vi "Sim_Yoke_Shin_TP059851_SPCC_Assignment.vi"() -> ()   [LabVIEW 2020]
uses:
  EnumControl.ctl
panel:
  in  "Enter":bool
  in  "User Input":string
  in  "Card Simulator":bool
  in  "Right Buttons":T1
  out "Right Menu":T2
  in  "Left Buttons":T3
  out "Left Menu":T4
  out "ATM Messages":string
  out "User ID":string
  out "Main Menu message":string
  out "Login":errorcluster
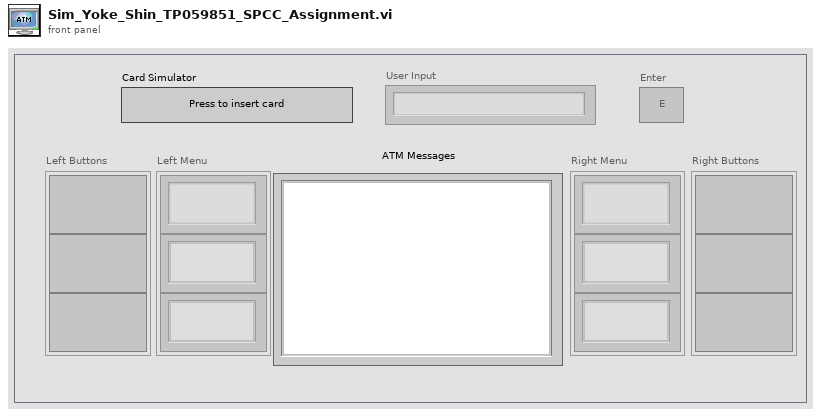
[diagram p1: front panel]
types:
  T1 = cluster{"Right 1 btn":bool, "Right 2 btn":bool, "Right 3 btn":bool}
  T2 = cluster{"Right 1 lbl":string, "Right 2 lbl":string, "Right 3 lbl":string}
  T3 = cluster{"Left 1 btn":bool, "Left 2 btn":bool, "Left 3 btn":bool}
  T4 = cluster{"Left 1 lbl":string, "Left 2 lbl":string, "Left 3 lbl":string}
  T5 = typedef "EnumControl.ctl" = enum16{"Idle", "Insert card", "Login click", "Validate Account", "Active Main Page", "Menu btn event", "Balance", "Deposit", "Withdraw", "Fast Cash", "Terminate"}
  T6 = enum8{"Enabled", "Disabled", "Disabled and Grayed Out"}
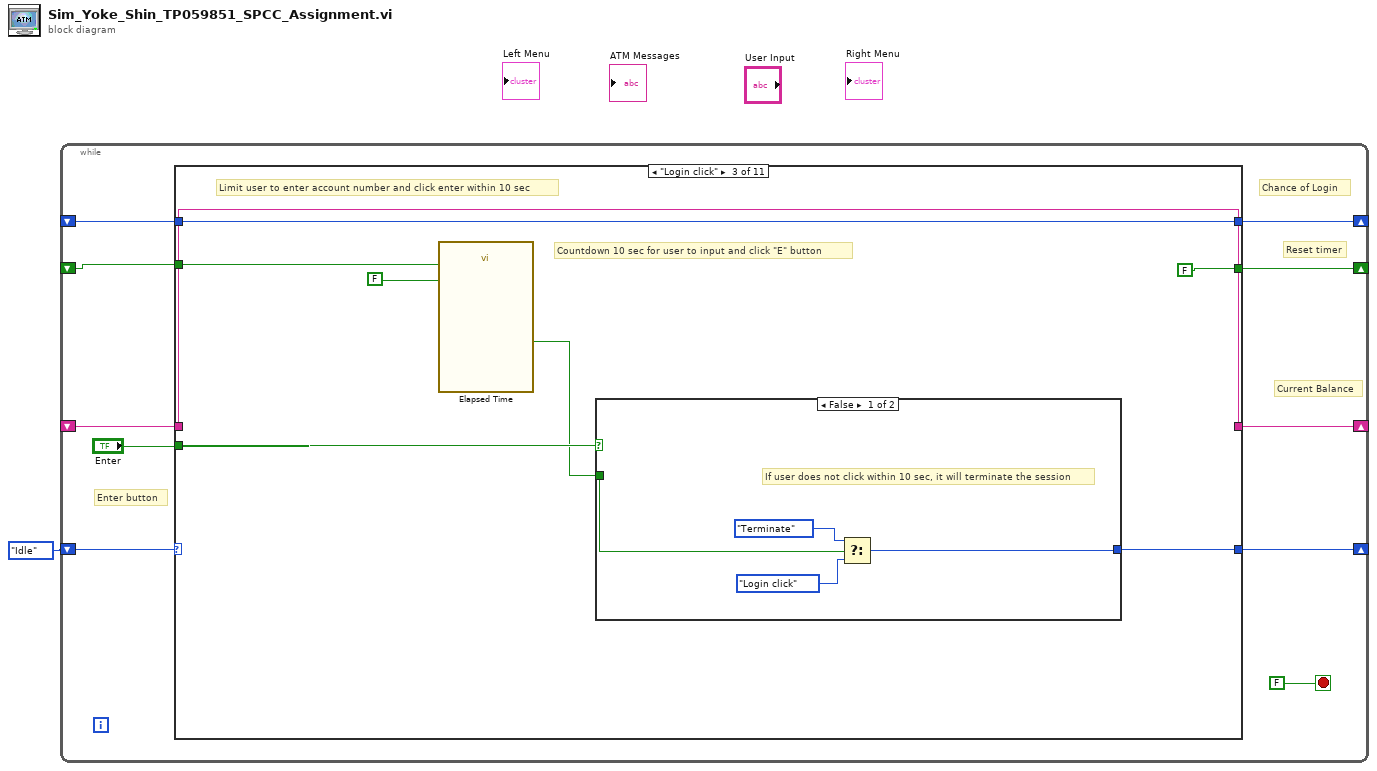
[diagram p0: block diagram]
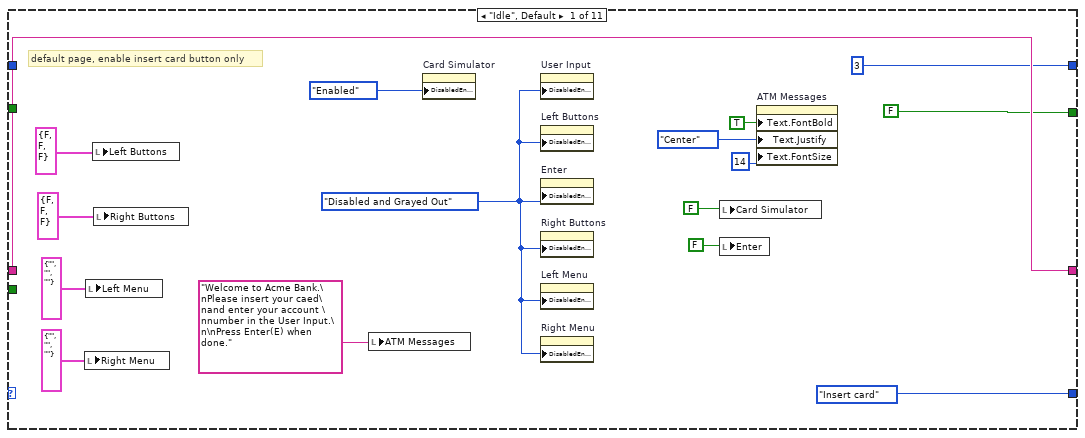
[diagram p2: hidden frame]
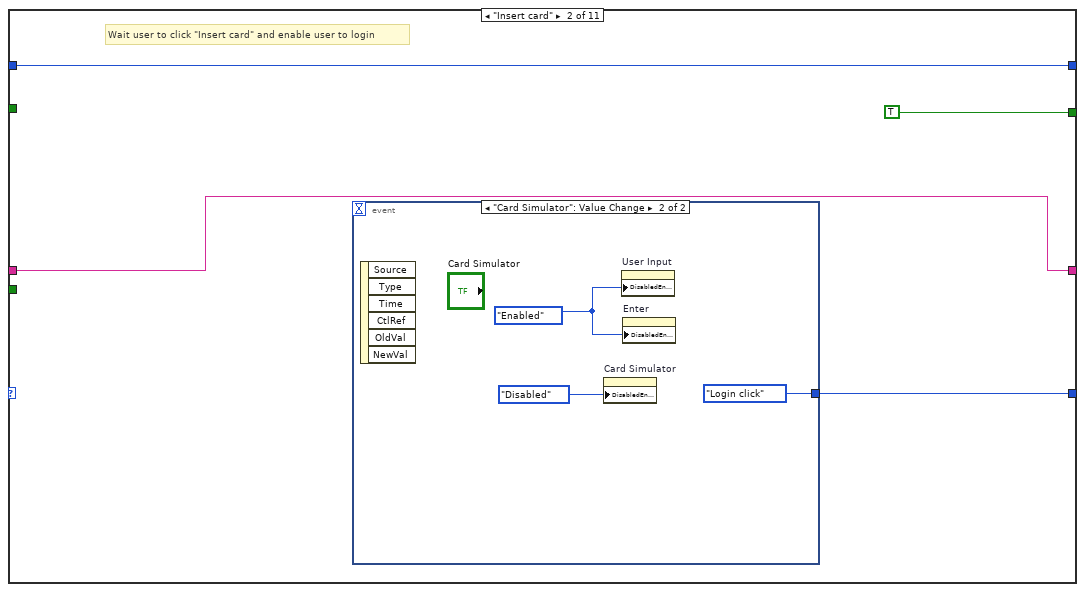
[diagram p3: hidden frame]
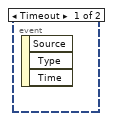
[diagram p4: hidden frame]
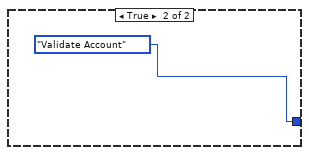
[diagram p5: hidden frame]
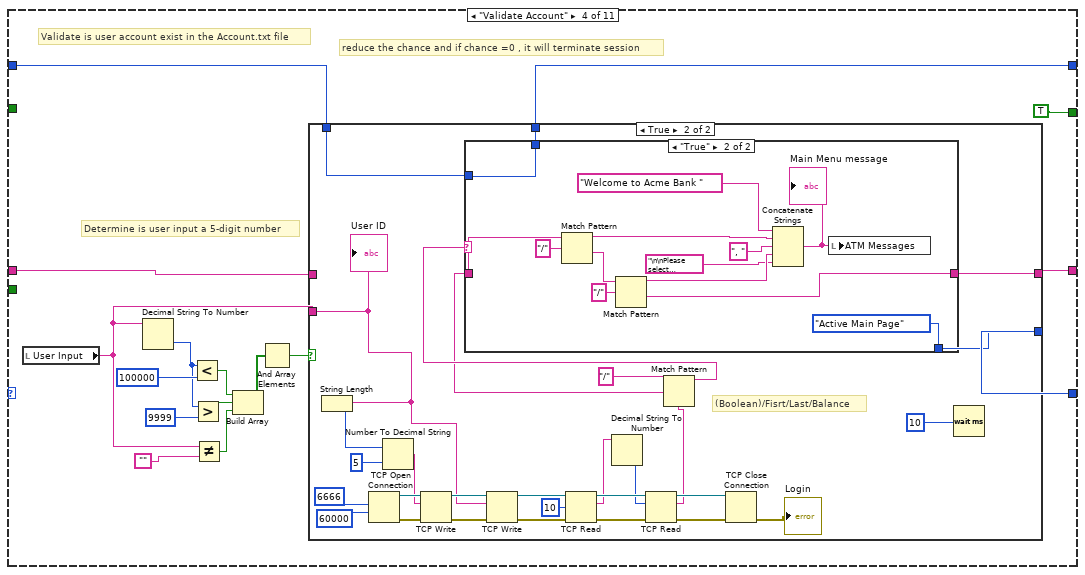
[diagram p6: hidden frame]
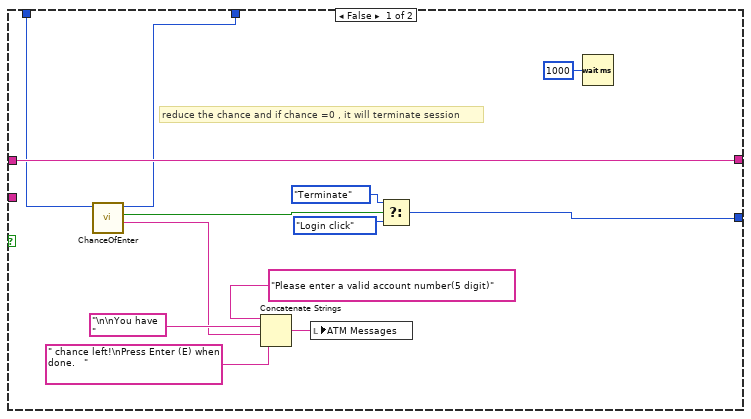
[diagram p7: hidden frame]
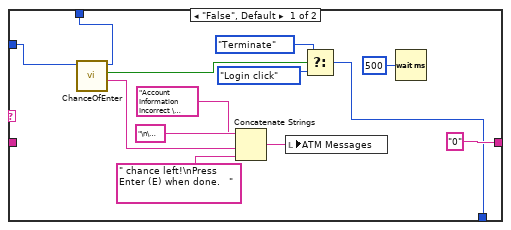
[diagram p8: hidden frame]
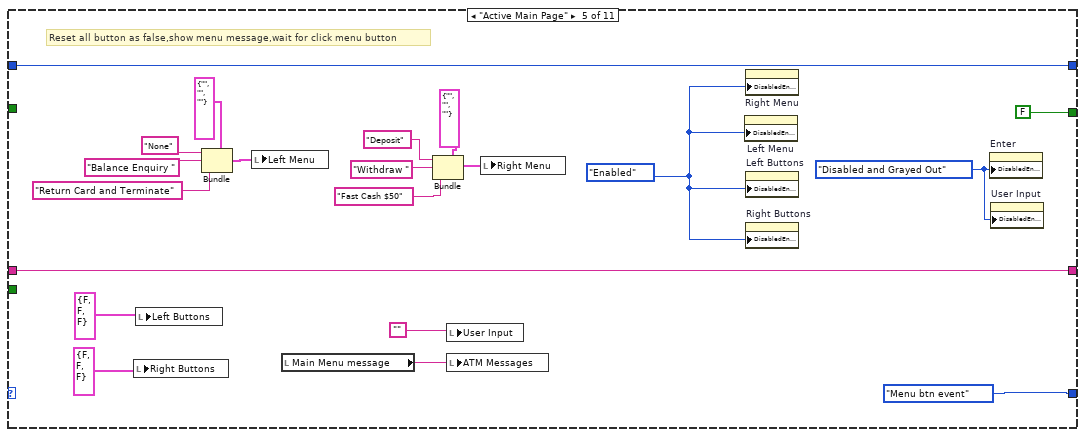
[diagram p9: hidden frame]
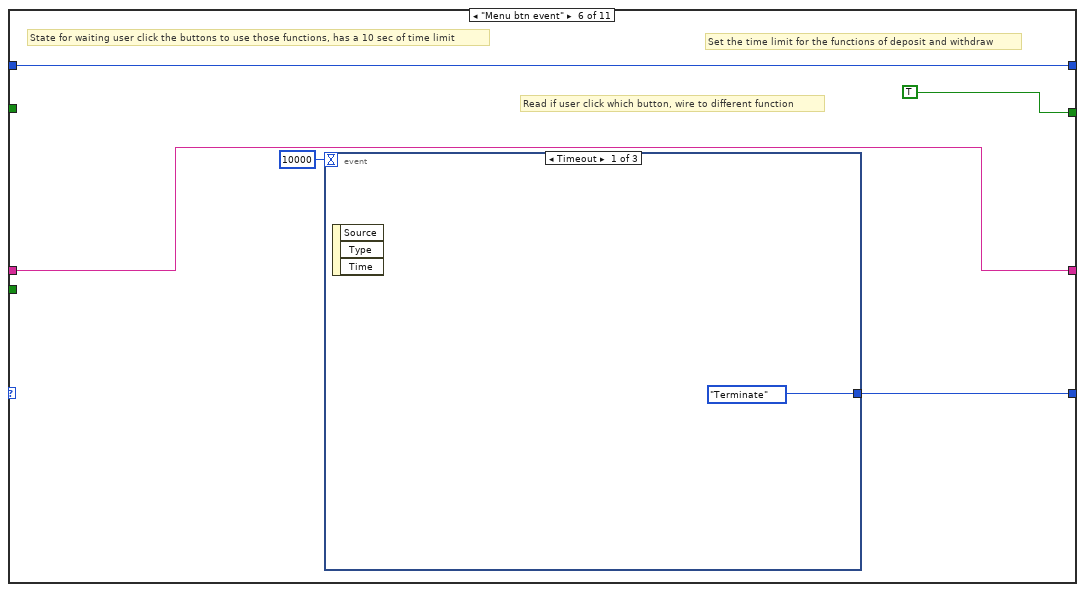
[diagram p10: hidden frame]
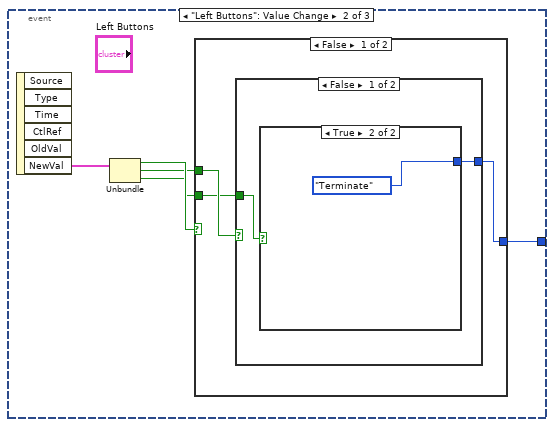
[diagram p11: hidden frame]
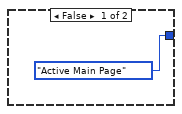
[diagram p12: hidden frame]
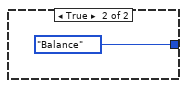
[diagram p13: hidden frame]
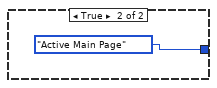
[diagram p14: hidden frame]
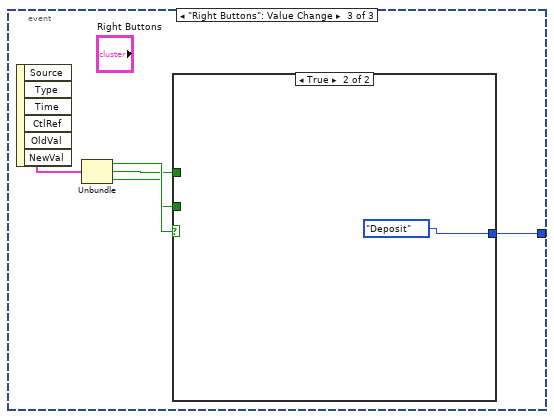
[diagram p15: hidden frame]
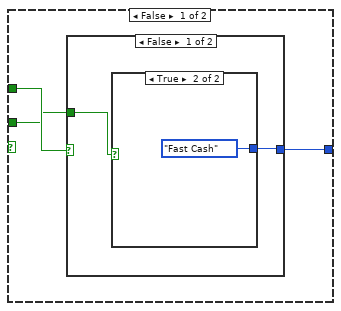
[diagram p16: hidden frame]
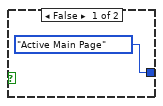
[diagram p17: hidden frame]
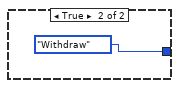
[diagram p18: hidden frame]
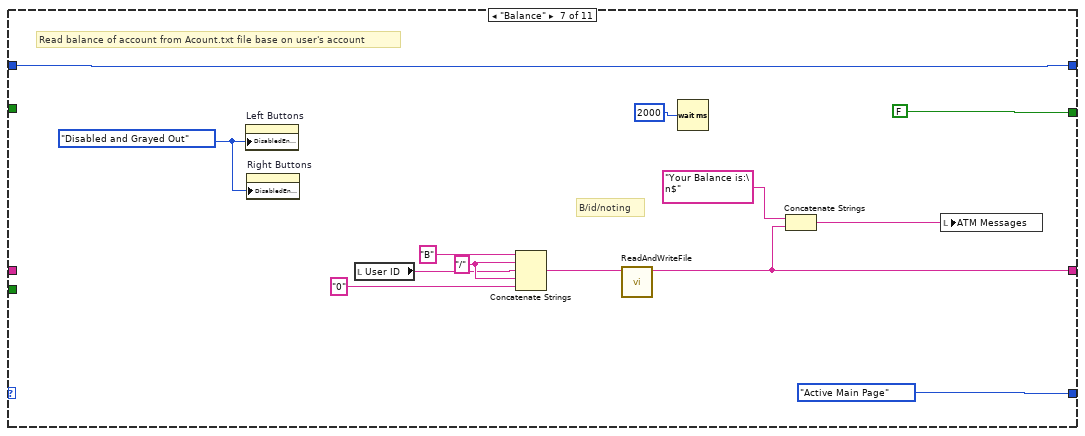
[diagram p19: hidden frame]
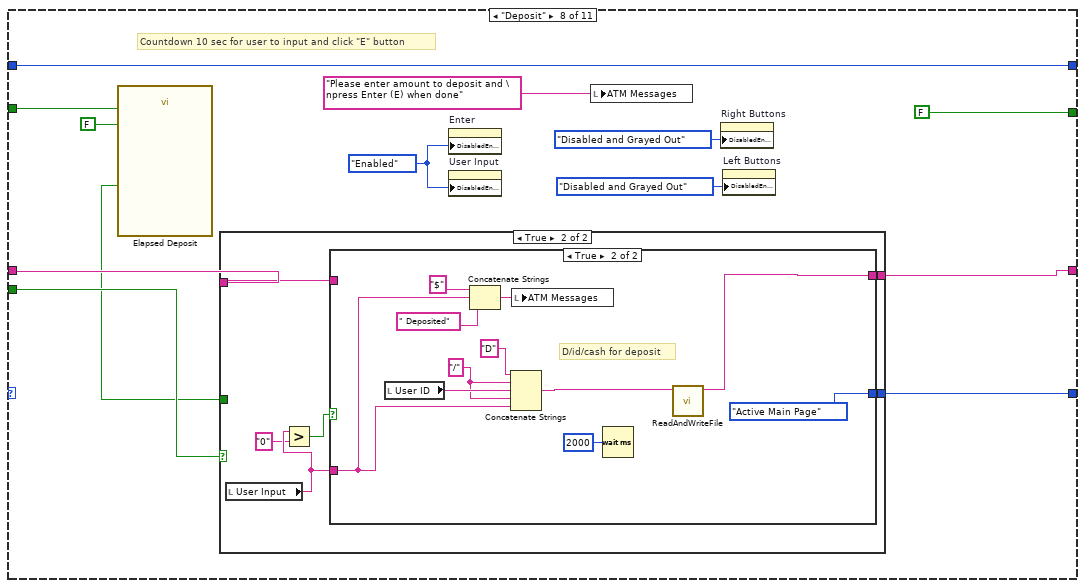
[diagram p20: hidden frame]
diagram:
  n1 = while {
    shift-right: [w9] -> _
    shift-left: EnumControl."Idle" ("Enum") -> [w11]
    shift-right: [w7] -> _
    shift-left: _ -> [w8]
    shift-right: [w4] -> _
    shift-left: _ -> [w5]
    shift-right: [w3] -> _
    shift-left: _ -> [w2]
    stop <- FALSE stop-if-true
    # "Enter button"
    # "Reset timer"
    # "Chance of Login"
    # "Current Balance"
    n2 = case shown="\"Login click\"" w11 {
      tunnel: [EnumControl."Insert card" ("Enum") w31 w41 w63 EnumControl."Menu btn event" ("Enum") w156 EnumControl."Active Main Page" ("Enum") w211 w250 w299 EnumControl."Idle" ("Enum")] -> w9
      tunnel: "Enter" -> [_ _ w42 _ _ _ _ w209 w248 _ _]
      tunnel: [w15 w30 w40 w62 w135 w155 w186 w206 w245 w297 w328] -> w7
      tunnel: w8 -> [w15 w30 w40 w55 w135 w155 _ w207 w246 w294 w328]
      tunnel: w5 -> [_ _ w37 _ _ _ _ w201 w240 _ _]
      tunnel: [FALSE TRUE FALSE TRUE FALSE TRUE FALSE FALSE FALSE FALSE FALSE] -> w4
      tunnel: [3 w28 w35 w60 w133 w152 w189 w199 w238 w295 3] -> w3
      tunnel: w2 -> [_ w28 w35 w61 w133 w152 w189 w199 w238 w295 _]
      frame "Idle", Default {
        w18 = T6."Disabled and Grayed Out" ("Disabled")
        # "default page, enable insert card button only"
        n3 = local write "Right Menu"(T2 {"Right 1 lbl"="", "Right 2 lbl"="", "Right 3 lbl"=""} ("right lbl")) -> ()
        n4 = local write "Left Menu"(T4 {"Left 1 lbl"="", "Left 2 lbl"="", "Left 3 lbl"=""} ("left lbl")) -> ()
        n5 = local write "Left Buttons"(T3 {"Left 1 btn"=FALSE, "Left 2 btn"=FALSE, "Left 3 btn"=FALSE} ("Left btn")) -> ()
        n6 = local write "Right Buttons"(T1 {"Right 1 btn"=FALSE, "Right 2 btn"=FALSE, "Right 3 btn"=FALSE} ("right btn")) -> ()
        n7 = local write "ATM Messages"("Welcome to Acme Bank.\nPlease insert your caed\nand enter your account \nnumber in the User Input.\n\nPress Enter(E) when done." ("ATM Messages")) -> ()
        n8 = property on="Card Simulator" class="Bool (strict)"("DisabledEnum"=T6."Enabled" ("Disabled")) -> ()  [unwired: 2 in, 2 out]
        n9 = property on="User Input" class="Str"("DisabledEnum"=w18) -> ()  [unwired: 2 in, 2 out]
        n10 = property on="Left Buttons" class="Clust (strict)"("DisabledEnum"=w18) -> ()  [unwired: 2 in, 2 out]
        n11 = property on="Enter" class="Bool (strict)"("DisabledEnum"=w18) -> ()  [unwired: 2 in, 2 out]
        n12 = property on="Right Buttons" class="Clust (strict)"("DisabledEnum"=w18) -> ()  [unwired: 2 in, 2 out]
        n13 = property on="Left Menu" class="Clust (strict)"("DisabledEnum"=w18) -> ()  [unwired: 2 in, 2 out]
        n14 = property on="Right Menu" class="Clust (strict)"("DisabledEnum"=w18) -> ()  [unwired: 2 in, 2 out]
        n15 = local write "Card Simulator"(FALSE ("Card Simulator")) -> ()
        n16 = local write "Enter"(FALSE ("Enter")) -> ()
        n17 = property on="ATM Messages" class="Str"("Text.FontBold"=TRUE ("Text.Font:Bold"), "Text.Justify"=enum16{"Left", "Center", "Right"}."Center" ("Text.Justification"), "Text.FontSize"=u32 14 ("Text.Font:Size")) -> ()  [unwired: 2 in, 2 out]
      }
      frame "Insert card" {
        # "Wait user to click \"Insert card\" and enable user to login"
        n18 = event shown="[1] \"Card Simulator\": Value Change" {
          selector: _ -> [_ _]
          dyn-events: _ -> [_ _]
          timeout: _ -> [_ _]
          tunnel: [_ EnumControl."Login click" ("Enum")] -> w31
          event Timeout {
            n19 = event-data() -> ()  [unwired: 1 in, 3 out]
          }
          event "Card Simulator": Value Change {
            w34 = T6."Enabled" ("Disabled")
            n20 = event-data() -> ()  [unwired: 1 in, 6 out]
            n21 = property on="Card Simulator" class="Bool (strict)"("DisabledEnum"=T6."Disabled" ("Disabled")) -> ()  [unwired: 2 in, 2 out]
            n22 = property on="User Input" class="Str"("DisabledEnum"=w34) -> ()  [unwired: 2 in, 2 out]
            n23 = property on="Enter" class="Bool (strict)"("DisabledEnum"=w34) -> ()  [unwired: 2 in, 2 out]
          }
        }
      }
      frame "Login click" {
        # "Limit user to enter account number and click enter within 10 sec"
        # "Countdown 10 sec for user to input and click \"E\" button"
        n24 = call "Elapsed Time"("Reset"=w37, "Auto Reset"=FALSE) -> ("Time has Elapsed"=w39:bool)  [unwired: 10 in, 7 out]
        n25 = case shown="False" w42 {
          tunnel: [w44 EnumControl."Validate Account" ("Enum")] -> w41
          tunnel: w39 -> [w43 _]
          frame False {
            # "If user does not click within 10 sec, it will terminate the session"
            n26 = Select(t=EnumControl."Terminate" ("Enum"), s=w43, f=EnumControl."Login click" ("Enum")) -> (s? t:f=w44:T5)
          }
          frame True {
          }
        }
      }
      frame "Validate Account" {
        # "Validate is user account exist in the Account.txt file"
        # "Determine is user input a 5-digit number"
        # "reduce the chance and if chance =0 , it will terminate session"
        n27 = local read "User Input"() -> (w57:string)
        n28 = Decimal String To Number(string=w57) -> (number=w53:i32)  [unwired: 2 in, 1 out]
        n29 = Less?(x=w53, y=100000) -> (x < y?=w50:bool)
        n30 = Greater?(x=w53, y=9999) -> (0:w51:bool)
        n31 = Not Equal?(x=w57, y="") -> (x != y?=w52:bool)
        n32 = Build Array "Build Array"(w50, w51, w52) -> (w49:bool[])
        n33 = And Array Elements(Boolean array=w49) -> (logical AND=w48:bool)
        n34 = case shown="True" w48 {
          tunnel: w57 -> [_ w90]
          tunnel: [w70 w82] -> w63
          tunnel: [w69 w79] -> w62
          tunnel: w61 -> [w67 w78]
          tunnel: [w66 w77] -> w60
          tunnel: w55 -> [w69 _]
          frame False {
            # "reduce the chance and if chance =0 , it will terminate session"
            n35 = call "ChanceOfEnter.vi"("Numeric in"=w67) -> ("String"=w64:string, "Boolean"=w65:bool, "Numeric out"=w66:i32)  [unwired: 8 in]
            n36 = Concatenate Strings("Please enter a valid account number(5 digit)" ("ATM Messages"), "\n\nYou have " ("string"), w64, " chance left!\nPress Enter (E) when done.   " ("string")) -> (w76:string)
            n37 = local write "ATM Messages"(w76) -> ()
            n38 = Select(t=EnumControl."Terminate" ("Enum"), s=w65, f=EnumControl."Login click" ("Enum")) -> (s? t:f=w70:T5)
            n39 = Wait (ms)(milliseconds to wait=u32 1000) -> ()  [unwired: 1 out]
          }
          frame True {
            # "(Boolean)/Fisrt/Last/Balance"
            n40 = String Length(string=w90) -> (length=w92:i32)
            n41 = TCP Open Connection(remote port or service name=u16 6666, timeout ms (60000)=60000) -> (connection ID=w97:refnum<k5>, error out=w105:errorcluster)  [unwired: 3 in]
            n42 = Number To Decimal String(number=w92, width (-)=i16 5) -> (decimal integer string=w91:string)
            n43 = TCP Write(connection ID=w97, data in=w91, error in (no error)=w105) -> (connection ID out=w96:refnum<k5>, error out=w104:errorcluster)  [unwired: 1 in, 1 out]
            n44 = TCP Write(connection ID=w96, data in=w90, error in (no error)=w104) -> (connection ID out=w95:refnum<k5>, error out=w103:errorcluster)  [unwired: 1 in, 1 out]
            n45 = TCP Read(connection ID=w95, bytes to read=10, error in (no error)=w103) -> (connection ID out=w94:refnum<k5>, data out=w88:string, error out=w102:errorcluster)  [unwired: 2 in]
            n46 = Decimal String To Number(string=w88) -> (number=w87:i32)  [unwired: 2 in, 1 out]
            n47 = TCP Read(connection ID=w94, bytes to read=w87, error in (no error)=w102) -> (connection ID out=w93:refnum<k5>, data out=w86:string, error out=w101:errorcluster)  [unwired: 2 in]
            n48 = Match Pattern(string=w86, regular expression="/") -> (before substring=w84:string, after substring=w83:string)  [unwired: 1 in, 2 out]
            n49 = case shown="\"True\"" w84 {
              tunnel: w83 -> [_ w131]
              tunnel: [w106 EnumControl."Active Main Page" ("Enum")] -> w82
              tunnel: ["0" ("data out") w120] -> w79
              tunnel: w78 -> [w113 w119]
              tunnel: [w110 w119] -> w77
              frame "False", Default {
                n50 = call "ChanceOfEnter.vi"("Numeric in"=w113) -> ("String"=w112:string, "Boolean"=w109:bool, "Numeric out"=w110:i32)  [unwired: 8 in]
                n51 = Concatenate Strings("Account Information Incorrect \nPlease Re-Enter Account Number. " ("ATM Messages"), "\n\nYou have " ("string"), w112, " chance left!\nPress Enter (E) when done.   " ("string")) -> (w116:string)
                n52 = local write "ATM Messages"(w116) -> ()
                n53 = Select(t=EnumControl."Terminate" ("Enum"), s=w109, f=EnumControl."Login click" ("Enum")) -> (s? t:f=w106:T5)
                n54 = Wait (ms)(milliseconds to wait=u32 500) -> ()  [unwired: 1 out]
              }
              frame "True" {
                n55 = Match Pattern(string=w131, regular expression="/") -> (before substring=w123:string, after substring=w125:string)  [unwired: 1 in, 2 out]
                n56 = Match Pattern(string=w125, regular expression="/") -> (before substring=w122:string, after substring=w120:string)  [unwired: 1 in, 2 out]
                n57 = Concatenate Strings("Welcome to Acme Bank " ("string"), w123, ", " ("string"), w122, "\n\nPlease select transaction by using the buttons. " ("string")) -> (w127:string)
                "Main Menu message" <- w127
                n58 = local write "ATM Messages"(w127) -> ()
              }
            }
            n59 = TCP Close Connection(connection ID=w93, error in (no error)=w101) -> (error out=→"Login":errorcluster)  [unwired: 1 in, 1 out]
            n60 = Wait (ms)(milliseconds to wait=u32 10) -> ()  [unwired: 1 out]
            "User ID" <- w90
          }
        }
      }
      frame "Active Main Page" {
        w141 = T6."Disabled and Grayed Out" ("Disabled")
        w138 = T6."Enabled" ("Disabled")
        # "Reset all button as false,show menu message,wait for click menu button"
        n61 = local write "Right Buttons"(T1 {"Right 1 btn"=FALSE, "Right 2 btn"=FALSE, "Right 3 btn"=FALSE} ("right btn")) -> ()
        n62 = local write "Left Buttons"(T3 {"Left 1 btn"=FALSE, "Left 2 btn"=FALSE, "Left 3 btn"=FALSE} ("Left btn")) -> ()
        n63 = Bundle(cluster=T2 {"Right 1 lbl"="", "Right 2 lbl"="", "Right 3 lbl"=""}, "Right 1 lbl"="None", "Right 2 lbl"="Balance Enquiry ", "Right 3 lbl"="Return Card and Terminate") -> (w147:T2)
        n64 = local write "Left Menu"(w147) -> ()
        n65 = local read "Main Menu message"() -> (w151:string)
        n66 = Bundle(cluster=T2 {"Right 1 lbl"="", "Right 2 lbl"="", "Right 3 lbl"=""}, "Right 1 lbl"="Deposit", "Right 2 lbl"="Withdraw ", "Right 3 lbl"="Fast Cash $50") -> (w142:T2)
        n67 = local write "User Input"("") -> ()
        n68 = local write "ATM Messages"(w151) -> ()
        n69 = local write "Right Menu"(w142) -> ()
        n70 = property on="Left Menu" class="Clust (strict)"("DisabledEnum"=w138) -> ()  [unwired: 2 in, 2 out]
        n71 = property on="Right Menu" class="Clust (strict)"("DisabledEnum"=w138) -> ()  [unwired: 2 in, 2 out]
        n72 = property on="Left Buttons" class="Clust (strict)"("DisabledEnum"=w138) -> ()  [unwired: 2 in, 2 out]
        n73 = property on="Right Buttons" class="Clust (strict)"("DisabledEnum"=w138) -> ()  [unwired: 2 in, 2 out]
        n74 = property on="Enter" class="Bool (strict)"("DisabledEnum"=w141) -> ()  [unwired: 2 in, 2 out]
        n75 = property on="User Input" class="Str"("DisabledEnum"=w141) -> ()  [unwired: 2 in, 2 out]
      }
      frame "Menu btn event" {
        # "State for waiting user click the buttons to use those functions, has a 10 sec of time limit"
        # "Set the time limit for the functions of deposit and withdraw"
        # "Read if user click which button, wire to different function"
        n76 = event shown="[0] Timeout" {
          selector: _ -> [_ _ _]
          dyn-events: _ -> [_ _ _]
          timeout: 10000 -> [_ _ _]
          tunnel: [EnumControl."Terminate" ("Enum") w160 w174] -> w156
          event Timeout {
            n77 = event-data() -> ()  [unwired: 1 in, 3 out]
          }
          event "Left Buttons": Value Change {
            n78 = event-data() -> ("NewVal"=w162:T3)  [unwired: 1 in, 5 out]
            n79 = Unbundle "Unbundle"(w162) -> ("Left 1 btn"=w161:bool, "Left 2 btn"=w159:bool, "Left 3 btn"=w158:bool)
            n80 = case shown="False" w161 {
              tunnel: [w164 EnumControl."Active Main Page" ("Enum")] -> w160
              tunnel: w159 -> [w165 _]
              tunnel: w158 -> [w163 _]
              frame False {
                n81 = case shown="False" w165 {
                  tunnel: [w166 EnumControl."Balance" ("Enum")] -> w164
                  tunnel: w163 -> [w167 _]
                  frame False {
                    n82 = case shown="True" w167 {
                      tunnel: [EnumControl."Active Main Page" ("Enum") EnumControl."Terminate" ("Enum")] -> w166
                      frame False {
                      }
                      frame True {
                      }
                    }
                  }
                  frame True {
                  }
                }
              }
              frame True {
              }
            }
          }
          event "Right Buttons": Value Change {
            n83 = event-data() -> ("NewVal"=w176:T1)  [unwired: 1 in, 5 out]
            n84 = Unbundle "Unbundle"(w176) -> ("Right 1 btn"=w175:bool, "Right 2 btn"=w173:bool, "Right 3 btn"=w172:bool)
            n85 = case shown="True" w175 {
              tunnel: [w178 EnumControl."Deposit" ("Enum")] -> w174
              tunnel: w173 -> [w179 _]
              tunnel: w172 -> [w177 _]
              frame False {
                n86 = case shown="False" w179 {
                  tunnel: [w180 EnumControl."Withdraw" ("Enum")] -> w178
                  tunnel: w177 -> [w181 _]
                  frame False {
                    n87 = case shown="True" w181 {
                      tunnel: [EnumControl."Active Main Page" ("Enum") EnumControl."Fast Cash" ("Enum")] -> w180
                      frame False {
                      }
                      frame True {
                      }
                    }
                  }
                  frame True {
                  }
                }
              }
              frame True {
              }
            }
          }
        }
      }
      frame "Balance" {
        w188 = T6."Disabled and Grayed Out" ("Disabled")
        w193 = "/" ("string")
        # "Read balance of account from Acount.txt file base on user's account"
        # "B/id/noting"
        n88 = property on="Left Buttons" class="Clust (strict)"("DisabledEnum"=w188) -> ()  [unwired: 2 in, 2 out]
        n89 = property on="Right Buttons" class="Clust (strict)"("DisabledEnum"=w188) -> ()  [unwired: 2 in, 2 out]
        n90 = local read "User ID"() -> (w192:string)
        n91 = Concatenate Strings("B" ("string"), w193, w192, w193, "0" ("string")) -> (w187:string)
        n92 = call "ReadAndWriteFile.vi"("String"=w187) -> ("data out"=w186:string)  [unwired: 10 in]
        n93 = Wait (ms)(milliseconds to wait=u32 2000) -> ()  [unwired: 1 out]
        n94 = Concatenate Strings("Your Balance is:\n$" ("ATM Messages"), w186) -> (w195:string)
        n95 = local write "ATM Messages"(w195) -> ()
      }
      frame "Deposit" {
        w210 = T6."Enabled" ("Disabled")
        # "Countdown 10 sec for user to input and click \"E\" button"
        n96 = call "Elapsed Deposit"("Reset"=w201, "Auto Reset"=FALSE) -> ("Time has Elapsed"=w200:bool)  [unwired: 10 in, 7 out]
        n97 = case shown="True" w209 {
          tunnel: [w212 w222] -> w211
          tunnel: w207 -> [w216 w221]
          tunnel: [w216 w220] -> w206
          tunnel: w200 -> [w215 _]
          frame False {
            n98 = Select(t=EnumControl."Terminate" ("Enum"), s=w215, f=EnumControl."Deposit" ("Enum")) -> (s? t:f=w212:T5)
          }
          frame True {
            n99 = local read "User Input"() -> (w219:string)
            n100 = Greater?(x=w219, y="0") -> (0:w217:bool)
            n101 = case shown="True" w217 {
              tunnel: [EnumControl."Active Main Page" ("Enum") EnumControl."Active Main Page" ("Enum")] -> w222
              tunnel: w221 -> [w224 _]
              tunnel: [w224 w227] -> w220
              tunnel: w219 -> [_ w228]
              frame False {
                n102 = Wait (ms)(milliseconds to wait=u32 1500) -> ()  [unwired: 1 out]
                n103 = local write "ATM Messages"("Please enter a valid amount!" ("ATM Messages")) -> ()
              }
              frame True {
                w233 = "/" ("string")
                # "D/id/cash for deposit"
                n104 = local read "User ID"() -> (w235:string)
                n105 = Concatenate Strings("$" ("string"), w228, " Deposited" ("string")) -> (w231:string)
                n106 = Concatenate Strings("D" ("string"), w233, w235, w233, w228) -> (w236:string)
                n107 = local write "ATM Messages"(w231) -> ()
                n108 = Wait (ms)(milliseconds to wait=u32 2000) -> ()  [unwired: 1 out]
                n109 = call "ReadAndWriteFile.vi"("String"=w236) -> ("data out"=w227:string)  [unwired: 10 in]
              }
            }
          }
        }
        n110 = property on="Enter" class="Bool (strict)"("DisabledEnum"=w210) -> ()  [unwired: 2 in, 2 out]
        n111 = property on="User Input" class="Str"("DisabledEnum"=w210) -> ()  [unwired: 2 in, 2 out]
        n112 = local write "ATM Messages"("Please enter amount to deposit and \npress Enter (E) when done" ("ATM Messages")) -> ()
        n113 = property on="Right Buttons" class="Clust (strict)"("DisabledEnum"=T6."Disabled and Grayed Out" ("Disabled")) -> ()  [unwired: 2 in, 2 out]
        n114 = property on="Left Buttons" class="Clust (strict)"("DisabledEnum"=T6."Disabled and Grayed Out" ("Disabled")) -> ()  [unwired: 2 in, 2 out]
      }
      frame "Withdraw" {
        w249 = T6."Enabled" ("Disabled")
        # "make sure input is valid and change the string to numeric"
        # "Countdown 10 sec for user to input and click \"E\" button"
        n115 = call "Elapsed Withdraw"("Reset"=w240, "Auto Reset"=FALSE) -> ("Time has Elapsed"=w239:bool)  [unwired: 10 in, 7 out]
        n116 = case shown="True" w248 {
          tunnel: [w251 w262] -> w250
          tunnel: w246 -> [w255 w260]
          tunnel: [w255 w261] -> w245
          tunnel: w239 -> [w254 _]
          frame False {
            n117 = Select(t=EnumControl."Terminate" ("Enum"), s=w254, f=EnumControl."Withdraw" ("Enum")) -> (s? t:f=w251:T5)
          }
          frame True {
            n118 = local read "User Input"() -> (w259:string)
            n119 = call "AvoidTypeZeroOrLesser.vi"("User Input"=w259, "data in"=w260) -> ("Boolean"=w258:bool, "Numeric"=w256:i32, "Numeric 2"=w257:i32)  [unwired: 7 in]
            n120 = case shown="True" w258 {
              tunnel: [EnumControl."Active Main Page" ("Enum") w273] -> w262
              tunnel: w259 -> [_ w272]
              tunnel: [w263 w270] -> w261
              tunnel: w260 -> [w263 w269]
              tunnel: w256 -> [_ w268]
              tunnel: w257 -> [_ w267]
              frame False {
                n121 = Wait (ms)(milliseconds to wait=u32 1500) -> ()  [unwired: 1 out]
                n122 = local write "ATM Messages"("Please enter a valid amount!" ("ATM Messages")) -> ()
              }
              frame True {
                # "is current balance greater or equal to user input"
                n123 = Greater Or Equal?(x=w267, y=w268) -> (x >= y?=w271:bool)
                n124 = case shown="False" w271 {
                  tunnel: [EnumControl."Active Main Page" ("Enum") EnumControl."Active Main Page" ("Enum")] -> w273
                  tunnel: w272 -> [_ w281]
                  tunnel: [w275 w278] -> w270
                  tunnel: w267 -> [_ _]
                  tunnel: w268 -> [_ _]
                  tunnel: w269 -> [w275 _]
                  frame False {
                    n125 = Wait (ms)(milliseconds to wait=u32 2000) -> ()  [unwired: 1 out]
                    n126 = local write "ATM Messages"("Insufficient funds in account \nPlease check your balance and try again " ("ATM Messages")) -> ()
                  }
                  frame True {
                    w282 = "/" ("string")
                    # "Open connection to server and pass the value of user input"
                    # "W/id/withdraw amount"
                    n127 = local read "User ID"() -> (w287:string)
                    n128 = Concatenate Strings("$" ("string"), w281, " Withdrawn" ("string")) -> (w286:string)
                    n129 = local write "ATM Messages"(w286) -> ()
                    n130 = Concatenate Strings("W" ("string"), w282, w287, w282, w281) -> (w279:string)
                    n131 = call "ReadAndWriteFile.vi"("String"=w279) -> ("data out"=w278:string)  [unwired: 10 in]
                    n132 = Wait (ms)(milliseconds to wait=u32 2000) -> ()  [unwired: 1 out]
                  }
                }
              }
            }
          }
        }
        n133 = property on="Enter" class="Bool (strict)"("DisabledEnum"=w249) -> ()  [unwired: 2 in, 2 out]
        n134 = property on="User Input" class="Str"("DisabledEnum"=w249) -> ()  [unwired: 2 in, 2 out]
        n135 = property on="Right Buttons" class="Clust (strict)"("DisabledEnum"=T6."Disabled and Grayed Out" ("Disabled")) -> ()  [unwired: 2 in, 2 out]
        n136 = property on="Left Buttons" class="Clust (strict)"("DisabledEnum"=T6."Disabled and Grayed Out" ("Disabled")) -> ()  [unwired: 2 in, 2 out]
        n137 = local write "ATM Messages"("Please enter amount to withdraw \nand press Enter (E) when done" ("ATM Messages")) -> ()
      }
      frame "Fast Cash" {
        w289 = T6."Disabled and Grayed Out" ("Disabled")
        # "make sure input is valid and change the string to numeric"
        # "Auto set user withdraw $50"
        n138 = local read "User Input"() -> (w293:string)
        n139 = call "AvoidTypeZeroOrLesser.vi"("User Input"=w293, "data in"=w294) -> ("Boolean"=w292:bool, "Numeric"=w290:i32, "Numeric 2"=w291:i32)  [unwired: 7 in]
        n140 = property on="User Input" class="Str"("DisabledEnum"=w289) -> ()  [unwired: 2 in, 2 out]
        n141 = property on="Right Buttons" class="Clust (strict)"("DisabledEnum"=w289) -> ()  [unwired: 2 in, 2 out]
        n142 = property on="Enter" class="Bool (strict)"("DisabledEnum"=w289) -> ()  [unwired: 2 in, 2 out]
        n143 = property on="Left Buttons" class="Clust (strict)"("DisabledEnum"=w289) -> ()  [unwired: 2 in, 2 out]
        n144 = case shown="True" w292 {
          tunnel: [EnumControl."Active Main Page" ("Enum") w310] -> w299
          tunnel: w293 -> [_ w309]
          tunnel: w291 -> [_ w307]
          tunnel: w290 -> [_ w306]
          tunnel: [w301 w308] -> w297
          tunnel: w294 -> [w301 w304]
          frame False {
            n145 = Wait (ms)(milliseconds to wait=u32 2000) -> ()  [unwired: 1 out]
            n146 = local write "ATM Messages"("Insufficient funds in account \nPlease check your balance and try again " ("ATM Messages")) -> ()
          }
          frame True {
            # "is current balance greater or equal to user input"
            n147 = Greater Or Equal?(x=w307, y=w306) -> (x >= y?=w305:bool)
            n148 = case shown="True" w305 {
              tunnel: [EnumControl."Active Main Page" ("Enum") EnumControl."Active Main Page" ("Enum")] -> w310
              tunnel: w309 -> [_ w318]
              tunnel: [w314 w315] -> w308
              tunnel: w304 -> [w314 _]
              frame False {
                n149 = Wait (ms)(milliseconds to wait=u32 1500) -> ()  [unwired: 1 out]
                n150 = local write "ATM Messages"("Insufficient funds in account \nPlease check your balance and try again " ("ATM Messages")) -> ()
              }
              frame True {
                w319 = "/" ("string")
                # "W/id/withdraw amount"
                # "Open connection to server and pass the value of user input"
                n151 = local read "User ID"() -> (w324:string)
                n152 = Concatenate Strings("$" ("string"), w318, " Withdrawn" ("string")) -> (w323:string)
                n153 = local write "ATM Messages"(w323) -> ()
                n154 = Concatenate Strings("W" ("string"), w319, w324, w319, w318) -> (w316:string)
                n155 = call "ReadAndWriteFile.vi"("String"=w316) -> ("data out"=w315:string)  [unwired: 10 in]
                n156 = Wait (ms)(milliseconds to wait=u32 2000) -> ()  [unwired: 1 out]
              }
            }
          }
        }
        n157 = local write "User Input"("50" ("User Input")) -> ()
      }
      frame "Terminate" {
        w330 = T6."Disabled and Grayed Out" ("Disabled")
        # "Terminate state, it will stay for 1.5 sec in this section and go to Idle state."
        n158 = local write "Card Simulator"(FALSE ("Card Simulator")) -> ()
        n159 = Wait (ms)(milliseconds to wait=u32 1500) -> ()  [unwired: 1 out]
        n160 = property on="Enter" class="Bool (strict)"("DisabledEnum"=w330) -> ()  [unwired: 2 in, 2 out]
        n161 = property on="User Input" class="Str"("DisabledEnum"=w330) -> ()  [unwired: 2 in, 2 out]
        n162 = local write "ATM Messages"("Your session has been terminated \ndue to inactivity or menu selection. \nPlease take your card \n\nGoodbye!  " ("ATM Messages")) -> ()
      }
    }
  }
